vi "MAIN  AJUSTE,ANALISIS,SIMULACION RPS.vi"() -> ()   [LabVIEW 2020]
panel:
  out "IR Película 2":dbl format="%#.4g"
  out "ángulo B valor medio":dbl
  out "otros ángulos cero":dbl[](array[numeric])
  in  "Stop":bool
  in  "Tab Control":T1(tab)
  in  "Extinction Coefficients":dbl[](array[slide]) step=0.01 scale=-5.0..5.0
  in  "Thicknesses (angstroms)":dbl[](array[slide]) step=5.0 scale=0.0..1000.0 scale format="%#.6g"
  in  "Refractive Indexes":dbl[](array[slide]) step=0.01 scale=1.0..5.0 scale format="%#.6g"
  out "q R theoretical":dbl format="%#.5g"
  in  "No.  Layers":u32=1
  in  "q maximum":dbl=89.0
  in  "q minimum":dbl=30.0
  in  "l(angstroms)":dbl=6328.0
  in  "Resolution":dbl=1000.0
  out "SPR Curve":cluster{"EJE X":dbl[], "EJE Y TEÓRICO":dbl[]}(graph)
  in  "No. Layers":u32=1
  in  "l(angstroms)":dbl=6328.0
  in  "Losses":dbl(slide)=0.9 step=0.001 scale=0.0..1.0 scale format="%#.6g"
  in  "Error":dbl(slide) step=0.01 scale=-5.0..5.0
  in  "Refractive Indexes":dbl[](array[slide]) step=0.001 scale=1.0..5.0 scale format="%#.6g"
  in  "Extinction Coefficients":dbl[](array[slide]) step=0.001 scale=-5.0..5.0 scale format="%#.6g"
  in  "Open File":path
  in  "Thicknesses (angstroms)":dbl[](array[slide]) scale=0.0..1000.0 scale format="%#.6g"
  out "CURVE FITTING":T2(graph)
  in  "Hacer ajuste":bool
  out "SPR Curve":cluster{"EJE X":dbl[], dbl[]}(graph)
  in  "q Final":dbl
  in  "q Starting":dbl
  in  "Open File":path
  in  "Realizar Análisis":bool
  out "qR":dbl
  out "Curve width":dbl format="%#.3g"
  out "q  Middle":dbl
  out "Minimun Intensity":dbl
  out "Maximum Intensity":dbl
  in  "Calcular ERROR":bool
  out "RI +error":dbl format="%#_4g"
  out "qB +error":dbl
  in  "Error (degrees)":dbl
  out "Refractive Index":dbl format="%#.4g"
  out "qB":dbl
  in  "Calcular":bool
  in  "q Final":dbl
  in  "q Starting":dbl
  in  "Open File":path
  out "Curve":cluster{dbl[], dbl[]}(graph)
  out "Curves":cluster{dbl[], dbl[]}[](graph)
  in  "q Final":dbl
  in  "q Starting":dbl
  in  "Open Film File":path
  in  "Open Substrate File":path
  in  "OK Button":bool
  out "Film RI":dbl format="%#.4g"
  out "Substrate RI":dbl format="%#.4g"
  out "Substrate qB":dbl
  out "Film qB":dbl
  in  "calcular error":bool
  in  "Error (degrees)":dbl
  out "Film qB +error":dbl
  out "Film RI +error":dbl format="%#.4g"
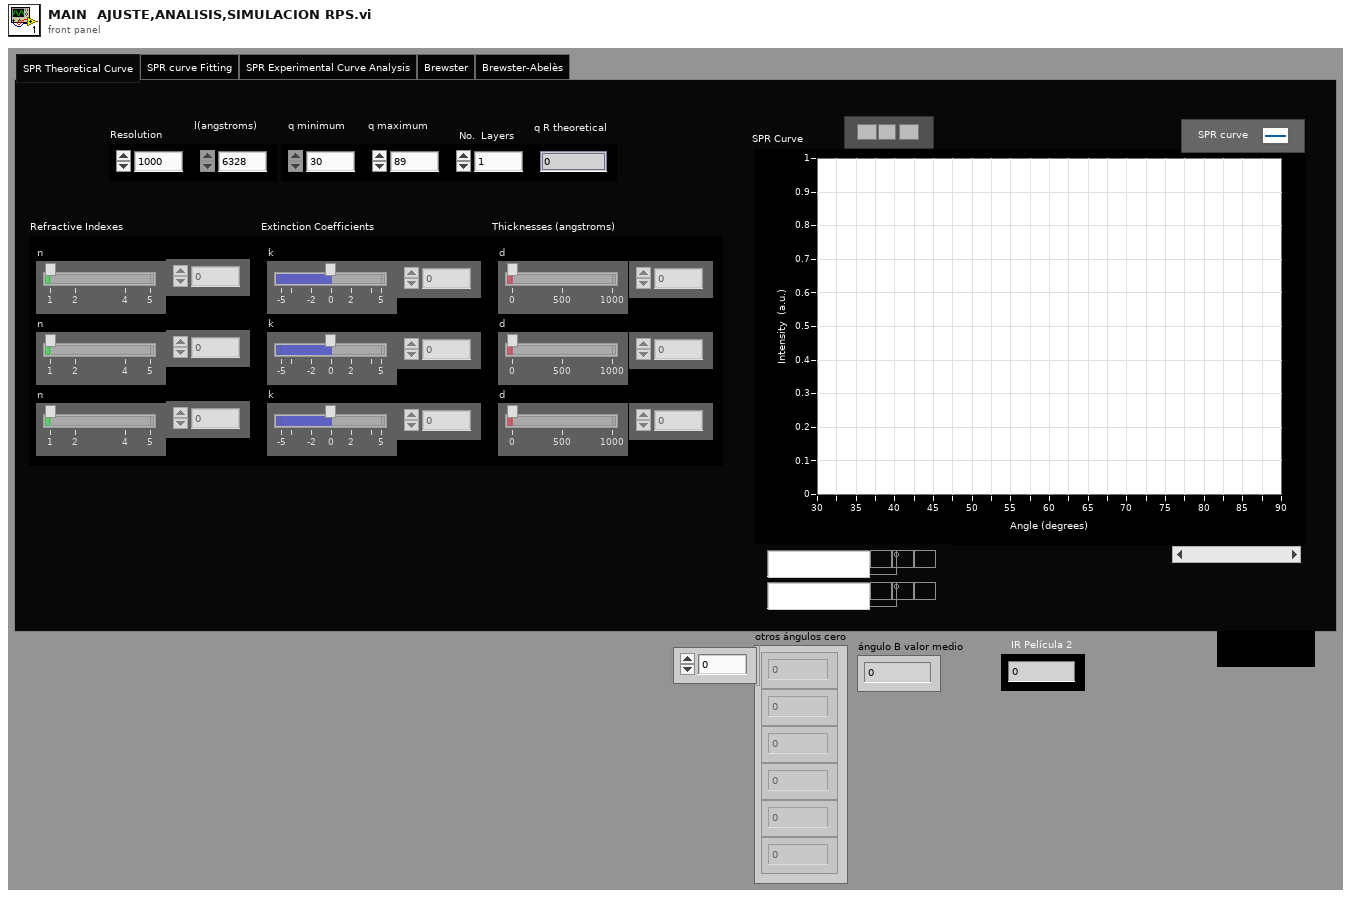
[diagram p1: front panel]
types:
  T1 = enum32{"SPR Theoretical Curve", "SPR curve Fitting", "SPR Experimental Curve Analysis", "Brewster", "Brewster-Abelès"}
  T2 = cluster{"EJE X":dbl[], "EJE Y NORMALIZADO":dbl[]}[]
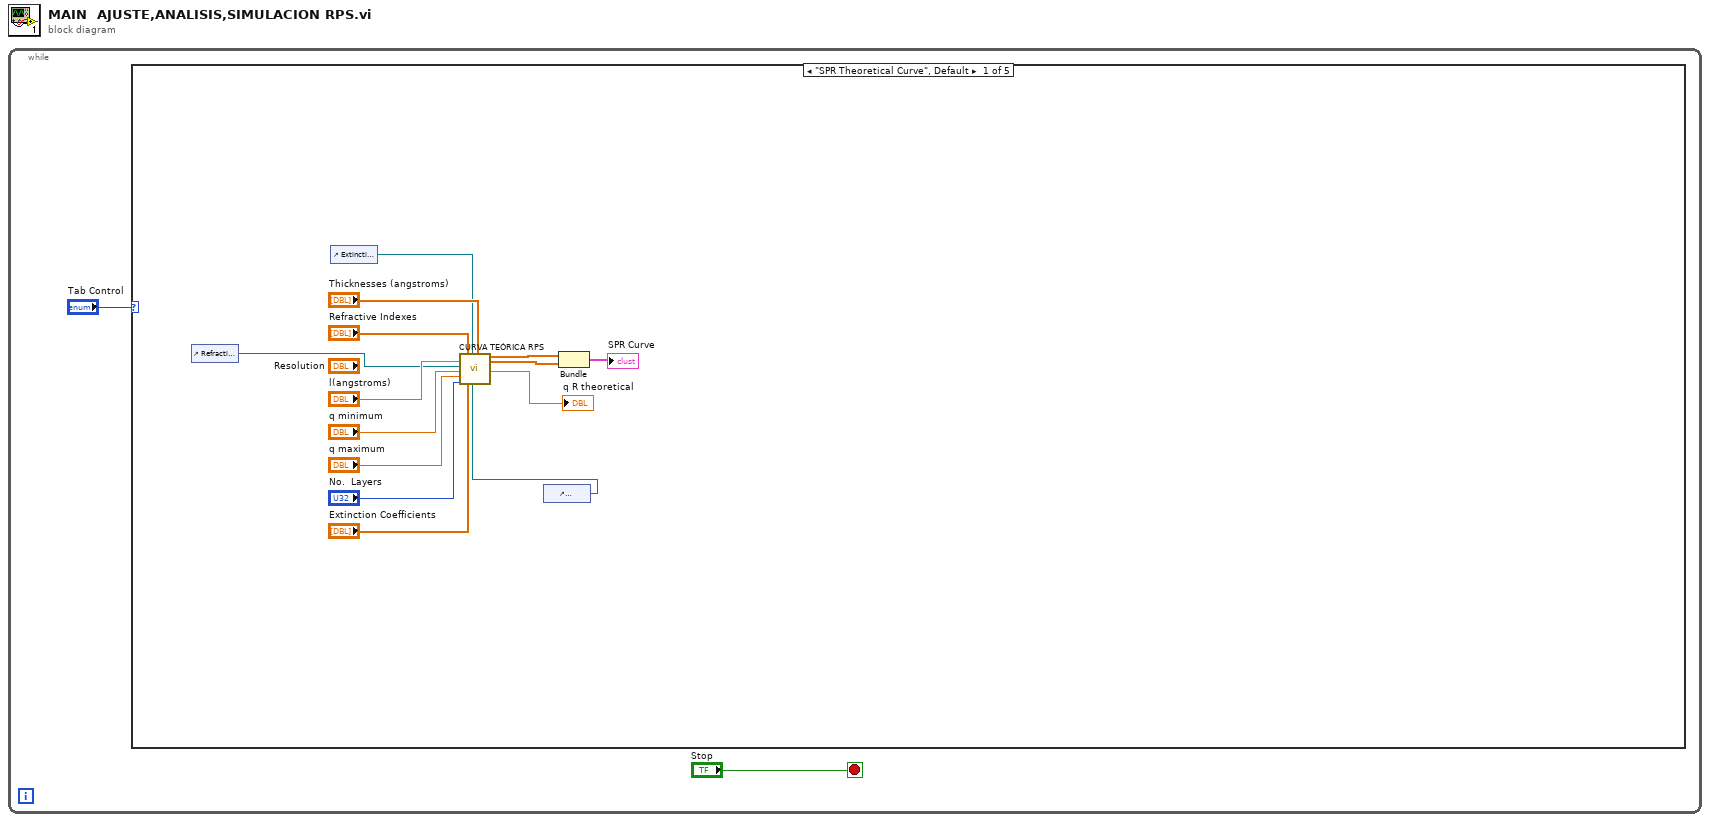
[diagram p0: block diagram]
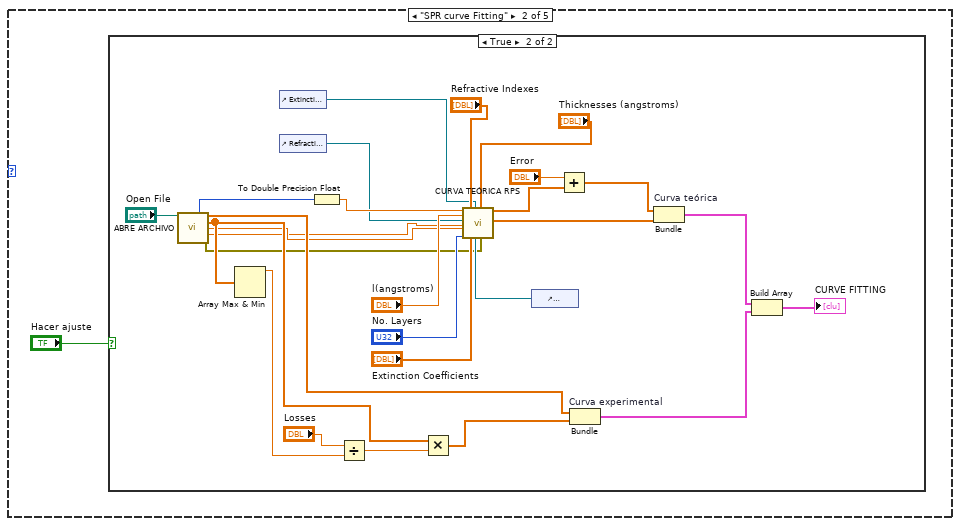
[diagram p2: hidden frame]
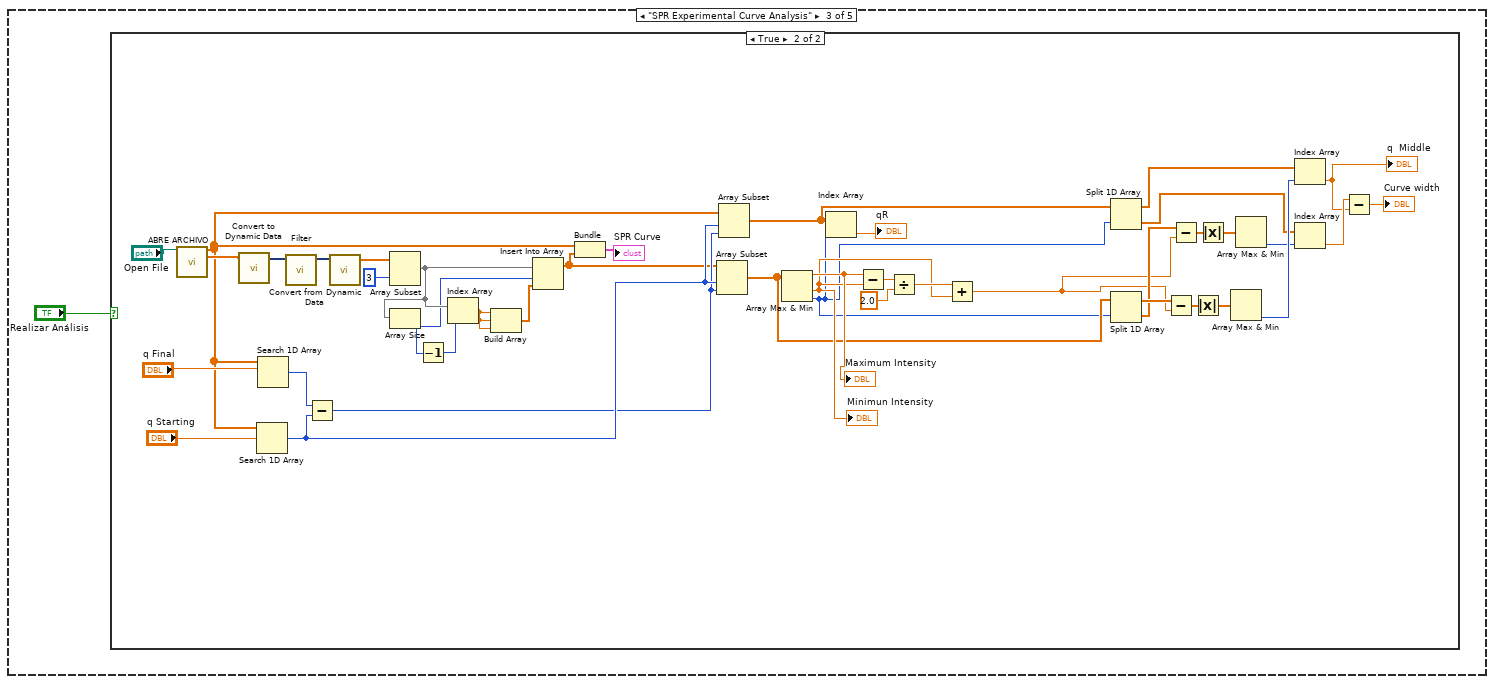
[diagram p4: hidden frame]
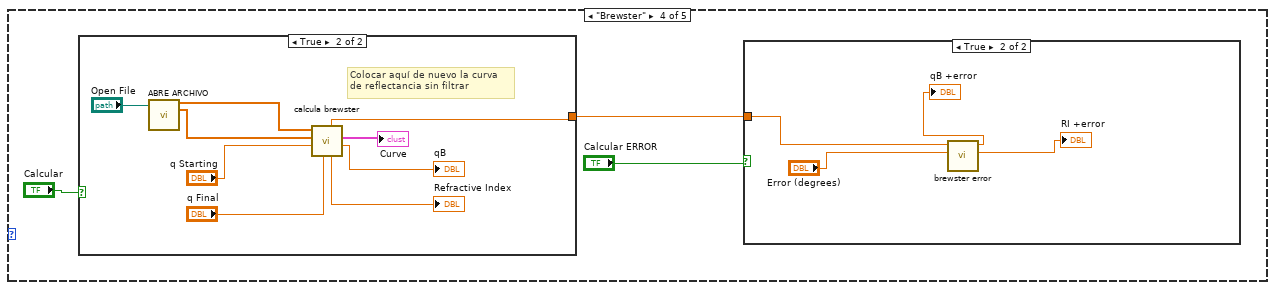
[diagram p6: hidden frame]
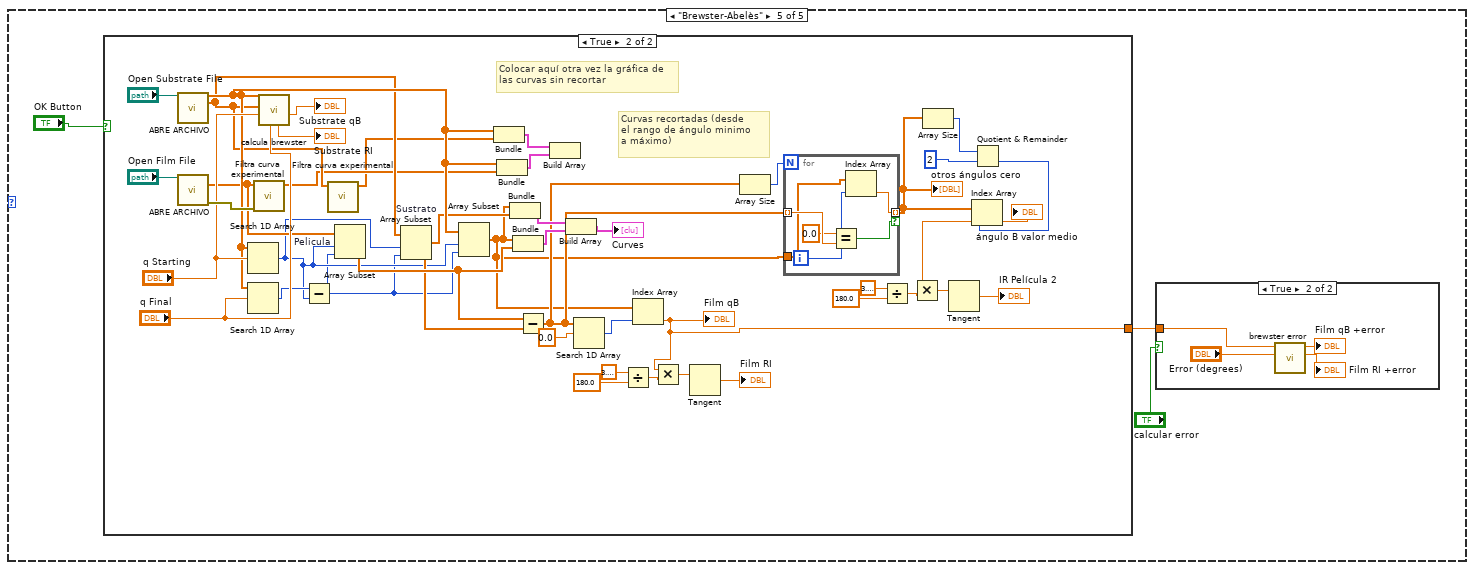
[diagram p9: hidden frame]
diagram:
  n1 = while {
    stop <- "Stop" stop-if-true
    n2 = case shown="\"SPR Theoretical Curve\", Default" "Tab Control" {
      frame "SPR Theoretical Curve", Default {
        n3 = control-ref of="Refractive Indexes"() -> (w4:refnum<vi>)
        n4 = control-ref of="Extinction Coefficients"() -> (w3:refnum<vi>)
        n5 = control-ref of="Thicknesses (angstroms)"() -> (w5:refnum<vi>)
        n6 = call "CURVA TEÓRICA RPS.vi"("l(angstroms)"="l(angstroms)", 2:"Índices de refracción"=w4, "q mínimo"="q minimum", "q máximo"="q maximum", "Número de capas"="No.  Layers", 6:"Índices de refracción"="Refractive Indexes", 7:"Coeficientes de extinción"="Extinction Coefficients", 8:"Coeficientes de extinción"=w3, "Espesores"=w5, "Espesores (angstroms)"="Thicknesses (angstroms)") -> ("EJE X"=w9:dbl[], "EJE Y TEÓRICO"=w8:dbl[], "q RPS teórico"=→"q R theoretical":dbl)  [unwired: 6 in, 1 out]
        n7 = Bundle("EJE X"=w9, "EJE Y TEÓRICO"=w8) -> (→"SPR Curve":cluster{"EJE X":dbl[], "EJE Y TEÓRICO":dbl[]})  [unwired: 1 in]
      }
      frame "SPR curve Fitting" {
        n8 = case shown="True" "Hacer ajuste" {
          frame False {
          }
          frame True {
            n9 = call "ABRE ARCHIVO.vi"("File Path Control"="Open File") -> ("Número de datos"=w23:i32, "EJE X"=w26:dbl[], "EJE Y"=w25:dbl[], "Ángulo máximo"=w24:dbl, "Ángulo mínimo"=w22:dbl, "error out"=w21:errorcluster)  [unwired: 9 in]
            n10 = Array Max & Min(array=w25) -> (max value=w40:dbl)  [unwired: 3 out]
            n11 = control-ref of="Extinction Coefficients"() -> (w19:refnum<vi>)
            n12 = control-ref of="Refractive Indexes"() -> (w29:refnum<vi>)
            n13 = To Double Precision Float(number=w23) -> (double precision float=w32:dbl)
            n14 = Divide(x="Losses", y=w40) -> (x/y=w39:dbl)
            n15 = Multiply(x=w25, y=w39) -> (x*y=w38:dbl[])
            n16 = control-ref of="Thicknesses (angstroms)"() -> (w28:refnum<vi>)
            n17 = call "CURVA TEÓRICA RPS.vi"("Resolución"=w32, "l(angstroms)"="l(angstroms)", 2:"Índices de refracción"=w29, "q mínimo"=w22, "q máximo"=w24, "Número de capas"="No. Layers", 6:"Índices de refracción"="Refractive Indexes", 7:"Coeficientes de extinción"="Extinction Coefficients", 8:"Coeficientes de extinción"=w19, "Espesores"=w28, "Espesores (angstroms)"="Thicknesses (angstroms)", "error in (no error)"=w21) -> ("EJE X"=w34:dbl[], "EJE Y TEÓRICO"=w33:dbl[])  [unwired: 4 in, 2 out]
            n18 = Add(x="Error", y=w34) -> (x+y=w42:dbl[])
            n19 = Bundle "Curva experimental"("EJE X"=w26, w38) -> (w18:cluster{"EJE X":dbl[], dbl[]})  [unwired: 1 in]
            n20 = Bundle "Curva teórica"(w42, "EJE Y TEÓRICO"=w33) -> (w27:cluster{dbl[], "EJE Y TEÓRICO":dbl[]})  [unwired: 1 in]
            n21 = Build Array(w27, w18) -> (→"CURVE FITTING":cluster{"EJE X":dbl[], "EJE Y TEÓRICO":dbl[]}[])
          }
        }
      }
      frame "SPR Experimental Curve Analysis" {
        n22 = case shown="True" "Realizar Análisis" {
          frame False {
          }
          frame True {
            n23 = call "ABRE ARCHIVO.vi"("File Path Control"="Open File") -> ("EJE X"=w70:dbl[], "EJE Y"=w80:dbl[])  [unwired: 9 in, 4 out]
            n24 = call "Convert to Dynamic Data"("Array"=w80) -> ("Dynamic Data Type"=w83:dynamicdata)  [unwired: 3 in]
            n25 = Search 1D Array(1D array=w70, element="q Starting") -> (index of element=w73:i32)  [unwired: 1 in]
            n26 = Search 1D Array(1D array=w70, element="q Final") -> (index of element=w84:i32)  [unwired: 1 in]
            n27 = call "Filter"("Signal"=w83) -> ("Filtered Signal"=w82:dynamicdata)  [unwired: 9 in, 1 out]
            n28 = Subtract(x=w84, y=w73) -> (x-y=w72:i32)
            n29 = call "Convert from Dynamic Data"("Dynamic Data Type"=w82) -> ("Array"=w74:dbl[])  [unwired: 3 in]
            n30 = Array Subset(array=w74, index=3 ("length")) -> (w79:dbl[])  [unwired: 1 in]
            n31 = Array Size(array=w79) -> (size(s)=w76:i32)
            n32 = Decrement(x=w76) -> (x-1=w78:i32)
            n33 = Index Array(array=w79, index=w78) -> (element=w77:dbl)
            n34 = Build Array(w77, w77, w77) -> (w75:dbl[])
            n35 = Insert Into Array(array=w79, index=w76, new element=w75) -> (w69:dbl[])
            n36 = Bundle("EJE X"=w70, w69) -> (→"SPR Curve":cluster{"EJE X":dbl[], dbl[]})  [unwired: 1 in]
            n37 = Array Subset(array=w69, index=w73, length=w72) -> (w62:dbl[])
            n38 = Array Subset(array=w70, index=w73, length=w72) -> (w58:dbl[])
            n39 = Array Max & Min(array=w62) -> (max value=w67:dbl, min value=w63:dbl, min index (indices)=w54:i32)  [unwired: 1 out]
            "Minimun Intensity" <- w63
            "Maximum Intensity" <- w67
            n40 = Index Array(array=w58, index=w54) -> (element=→"qR":dbl)
            n41 = Subtract(x=w67, y=w63) -> (x-y=w66:dbl)
            n42 = Divide(x=w66, y=2.0) -> (x/y=w64:dbl)
            n43 = Add(x=w64, y=w63) -> (x+y=w50:dbl)
            n44 = Split 1D Array(array=w58, index=w54) -> (first subarray=w57:dbl[], second subarray=w55:dbl[])
            n45 = Split 1D Array(array=w62, index=w54) -> (first subarray=w61:dbl[], second subarray=w51:dbl[])
            n46 = Subtract(x=w61, y=w50) -> (x-y=w60:dbl[])
            n47 = Subtract(x=w51, y=w50) -> (x-y=w52:dbl[])
            n48 = Absolute Value(x=w60) -> (abs(x)=w59:dbl[])
            n49 = Absolute Value(x=w52) -> (abs(x)=w53:dbl[])
            n50 = Array Max & Min(array=w59) -> (min index (indices)=w56:i32)  [unwired: 3 out]
            n51 = Array Max & Min(array=w53) -> (min index (indices)=w49:i32)  [unwired: 3 out]
            n52 = Index Array(array=w57, index=w56) -> (element=w47:dbl)
            "q  Middle" <- w47
            n53 = Index Array(array=w55, index=w49) -> (element=w48:dbl)
            n54 = Subtract(x=w48, y=w47) -> (x-y=→"Curve width":dbl)
          }
        }
      }
      frame "Brewster" {
        n55 = case shown="True" "Calcular" {
          tunnel: [_ w98] -> w88
          frame False {
          }
          frame True {
            # "Colocar aquí de nuevo la curva\nde reflectancia sin filtrar"
            n56 = call "ABRE ARCHIVO.vi"("File Path Control"="Open File") -> ("EJE X"=w100:dbl[], "EJE Y"=w99:dbl[])  [unwired: 9 in, 4 out]
            n57 = call "calcula brewster.vi"("Ángulo Final"="q Final", "Ángulo Inicial"="q Starting", "EJE Y"=w99, "EJE X"=w100) -> ("Ángulo de Brewster"=→"qB":dbl, "Curva FILTRADA"=→"Curve":cluster{dbl[], dbl[]}, "Índice de Refracción"=→"Refractive Index":dbl, "Numeric Control"=w98:dbl)  [unwired: 3 in, 1 out]
          }
        }
        n58 = case shown="True" "Calcular ERROR" {
          tunnel: w88 -> [_ w94]
          frame False {
          }
          frame True {
            n59 = call "brewster error.vi"("Error (grados)"="Error (degrees)", "Numeric Control"=w94) -> ("Índice de Refracción +error"=→"RI +error":dbl, "Ángulo de Brewster +error"=→"qB +error":dbl)  [unwired: 8 in]
          }
        }
      }
      frame "Brewster-Abelès" {
        n60 = case shown="True" "OK Button" {
          tunnel: [_ w128] -> w105
          frame False {
          }
          frame True {
            # "Curvas recortadas (desde\nel rango de ángulo minimo \na máximo)"
            # "Colocar aquí otra vez la gráfica de\nlas curvas sin recortar"
            n61 = call "ABRE ARCHIVO.vi"("File Path Control"="Open Substrate File") -> ("EJE X"=w134:dbl[], "EJE Y"=w132:dbl[])  [unwired: 9 in, 4 out]
            n62 = call "ABRE ARCHIVO.vi"("File Path Control"="Open Film File") -> ("EJE Y"=w133:dbl[], "error out"=w149:errorcluster)  [unwired: 9 in, 4 out]
            n63 = Search 1D Array(1D array=w134, element="q Starting") -> (index of element=w125:i32)  [unwired: 1 in]
            n64 = Search 1D Array(1D array=w134, element="q Final") -> (index of element=w146:i32)  [unwired: 1 in]
            n65 = call "Filtra curva experimental.vi"("error in (no error)"=w149, "Y"=w133) -> ("Y Filtrada"=w123:dbl[])  [unwired: 7 in, 2 out]
            n66 = call "calcula brewster.vi"("Ángulo Final"="q Final", "Ángulo Inicial"="q Starting", "EJE Y"=w132, "EJE X"=w134) -> ("Ángulo de Brewster"=→"Substrate qB":dbl, "Índice de Refracción"=→"Substrate RI":dbl)  [unwired: 3 in, 3 out]
            n67 = Subtract(x=w146, y=w125) -> (x-y=w124:i32)
            n68 = call "Filtra curva experimental.vi"("Y"=w132) -> ("Y Filtrada"=w122:dbl[])  [unwired: 8 in, 2 out]
            n69 = Array Subset "Pelicula"(array=w133, index=w125, length=w124) -> (w131:dbl[])
            n70 = Array Subset "Sustrato"(array=w132, index=w125, length=w124) -> (w130:dbl[])
            n71 = Array Subset(array=w134, index=w125, length=w124) -> (w121:dbl[])
            n72 = Bundle("EJE X"=w134, "Y Filtrada"=w122) -> (w142:cluster{"EJE X":dbl[], "Y Filtrada":dbl[]})  [unwired: 1 in]
            n73 = Bundle("EJE X"=w134, "Y Filtrada"=w123) -> (w143:cluster{"EJE X":dbl[], "Y Filtrada":dbl[]})  [unwired: 1 in]
            n74 = Bundle(w121, w130) -> (w129:cluster{dbl[], dbl[]})  [unwired: 1 in]
            n75 = Bundle(w121, w131) -> (w145:cluster{dbl[], dbl[]})  [unwired: 1 in]
            n76 = Subtract(x=w131, y=w130) -> (x-y=w126:dbl[])
            n77 = Build Array(w142, w143) -> ()  [unwired: 1 out]
            n78 = Build Array(w129, w145) -> (→"Curves":cluster{dbl[], dbl[]}[])
            n79 = Search 1D Array(1D array=w126, element=0.0) -> (index of element=w140:i32)  [unwired: 1 in]
            n80 = Divide(x=3.141592653589793, y=180.0) -> (x/y=w137:dbl)
            n81 = Index Array(array=w121, index=w140) -> (element=w128:dbl)
            "Film qB" <- w128
            n82 = Multiply(x=w128, y=w137) -> (x*y=w138:dbl)
            n83 = Tangent(1:w138) -> (0:→"Film RI":dbl)
            n84 = Array Size(array=w126) -> (size(s)=w127:i32)
            n85 = for {
              N: w127 -> [_]
              tunnel: w126 -> [w159] mode=indexing
              tunnel: [w154] -> w118 mode=indexing if=w157
              tunnel: w121 -> [w156]
              i -> [w155]
              n86 = Equal?(x=0.0, y=w159) -> (x = y?=w157:bool)
              n87 = Index Array(array=w156, index=w155) -> (element=w154:dbl)
            }
            "otros ángulos cero" <- w118
            n88 = Divide(x=3.141592653589793, y=180.0) -> (x/y=w117:dbl)
            n89 = Array Size(array=w118) -> (size(s)=w120:i32)
            n90 = Quotient & Remainder(x=w120, y=2) -> (floor(x/y)=w111:i32)  [unwired: 1 out]
            n91 = Index Array(array=w118, index=w111) -> (element=w114:dbl)
            "ángulo B valor medio" <- w114
            n92 = Multiply(x=w114, y=w117) -> (x*y=w112:dbl)
            n93 = Tangent(1:w112) -> (0:→"IR Película 2":dbl)
          }
        }
        n94 = case shown="True" "calcular error" {
          tunnel: w105 -> [_ w109]
          frame False {
          }
          frame True {
            n95 = call "brewster error.vi"("Error (grados)"="Error (degrees)", "Numeric Control"=w109) -> ("Índice de Refracción +error"=→"Film RI +error":dbl, "Ángulo de Brewster +error"=→"Film qB +error":dbl)  [unwired: 8 in]
          }
        }
      }
    }
  }
